vi "Check For Team.vi"(7 "Team Index":i32, 10 "Direction":T1, 11 "Map":i32[](array[numeric])) -> (3 "Clear?":bool)   [LabVIEW 2020, in "Common.lvlib"]
uses:
  Common.lvlib
  Type Defs/Direction Enum.ctl
  Type Defs/SB Type Defs.lvlib
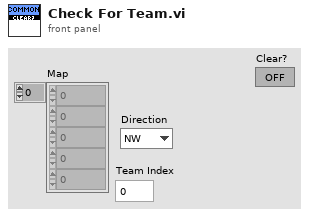
[diagram p1: front panel]
types:
  T1 = typedef "SB Type Defs.lvlib/Direction Enum.ctl" = enum16{"NW", "N", "NE", "E", "SE", "S", "SW", "W"}
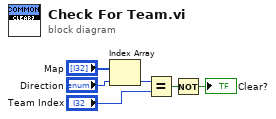
[diagram p0: block diagram]
diagram:
  n1 = Index Array(array="Map", index="Direction") -> (element=w3:i32)
  n2 = Equal?(x=w3, y="Team Index") -> (x = y?=w6:bool)
  n3 = Not(x=w6) -> (.not. x?=→"Clear?":bool)
